vi "Set Context.vi"(8 "error in (no error)":errorcluster, 10 "Process Context":refnum<class "Debug View.lvclass">, 11 "Process In":refnum<class "Debug View.lvclass">) -> (0 "error out":errorcluster, 3 "Process Out":refnum<class "Debug View.lvclass">)   [LabVIEW 2020]
doc: "Framework method for setting the context of a process. Any process added to an application automatically gets the correct context by the framework and using this method is not necessary."
uses:
  Debug View.lvclass
  Debug View.lvclass/Debug View.ctl
  <vilib>/Utility/error.llb/Clear Errors.vi
  <vilib>/Utility/error.llb/Error Cluster From Error Code.vi
  <vilib>/ErrorRing/Error Ring.xnode
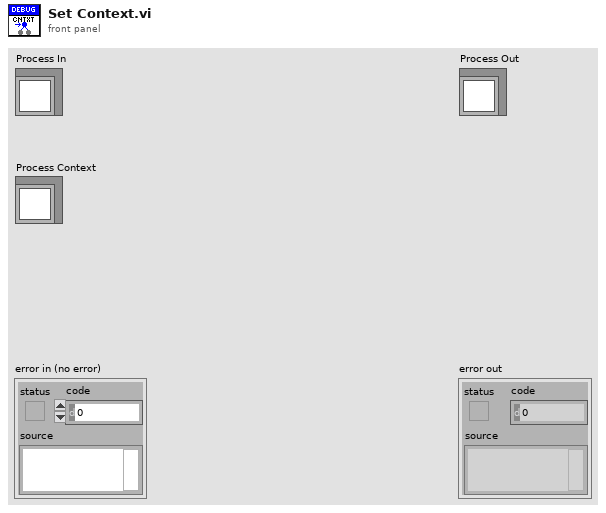
[diagram p1: front panel]
types:
  T1 = typedef "Lifecycle State.ctl" = enum16{"Uninitialized", "Initialized", "Started", "Running", "Stopped", "Finished"}
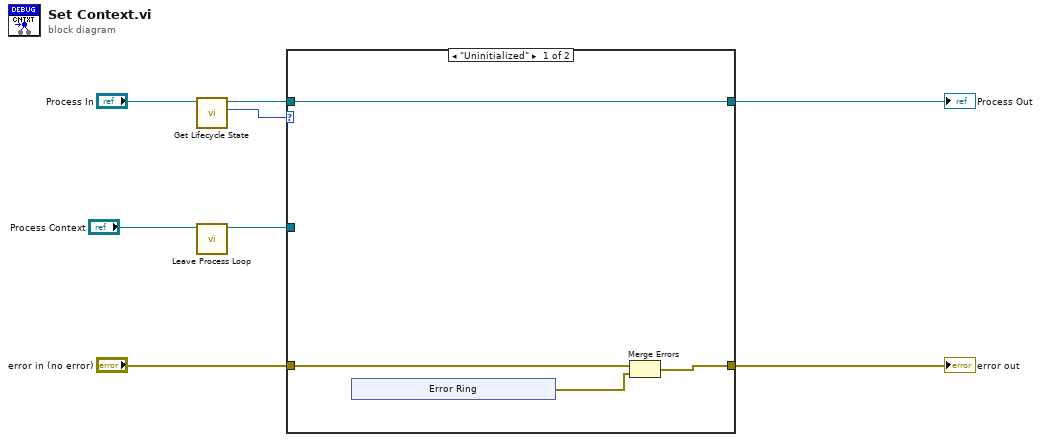
[diagram p0: block diagram]
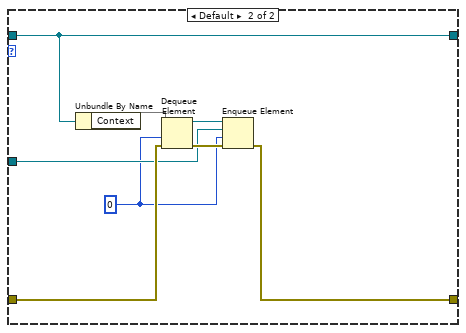
[diagram p2: hidden frame]
diagram:
  n1 = call "Get Lifecycle State.vi"("Process In"="Process In") -> ("Lifecycle State"=w3:T1, "Process Out"=w5:refnum<class "Debug View.lvclass">)  [unwired: 7 in, 2 out]
  n2 = call "Leave Process Loop.vi"("Process In"="Process Context") -> ("Process Out"=w2:refnum<class "Debug View.lvclass">)  [unwired: 9 in, 1 out]
  n3 = case shown="\"Uninitialized\"" w3 {
    tunnel: [w12 w24] -> w8
    tunnel: [w10 w20] -> w7
    tunnel: w2 -> [_ w18]
    tunnel: w5 -> [w12 w24]
    tunnel: "error in (no error)" -> [w11 w19]
    frame "Uninitialized" {
      n4 = xnode "Error Ring"() -> ("error out"=w9:errorcluster)
      n5 = Merge Errors(w11, w9) -> (w10:errorcluster)
    }
    frame Default {
      w17 = 0 ("timeout in ms (-1)")
      n6 = Unbundle By Name(w24) -> ("Context"=w23)
      n7 = Dequeue Element(queue=w23, timeout in ms (-1)=w17, error in (no error)=w19) -> (queue out=w22:refnum<queue>, error out=w21:errorcluster)  [unwired: 2 out]
      n8 = Enqueue Element(queue=w22, element=w18, timeout in ms (-1)=w17, error in (no error)=w21) -> (error out=w20:errorcluster)  [unwired: 2 out]
    }
  }
  "error out" <- w7
  "Process Out" <- w8
